vi "fxpProperty_OverflowModeDisabled_Write.vi"(4 "error in (no error)":errorcluster, 5 "Value":bool, 6 "Container State":T7, 7 "Display State In":T1) -> (0 "error out":errorcluster, 3 "Display State Out":T1)   [LabVIEW 2020, in "FXP.xctl"]
uses:
  <vilib>/fxp/FXPxcontrol/FXP.xctl
  <vilib>/_xctls/Container State.ctl
  <vilib>/fxp/FXPxcontrol/fxpState.ctl
  <vilib>/fxp/LVFixedPointQuantizationPolicyTypeDef.ctl
  <vilib>/fxp/LVFixedPointOverflowPolicyTypeDef.ctl
  <vilib>/fxp/FXPxcontrol/fxpChangeEvent.ctl
  <vilib>/fxp/FXPxcontrol/fxpValueChangeControl.ctl
  <vilib>/fxp/FXPxcontrol/fxpMixedStateStatus.ctl
  <vilib>/_xctls/XControlSupport.lvlib
panel:
  # "Replace the Value Control below with a Control of desired type.\nDo not remove this Control or the others from the connector pane.\nDo not change the connector pane pattern.\nThe Value control should always be the third terminal from top on the input side in the connector pane."
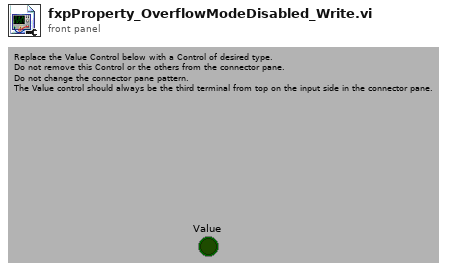
[diagram p1: front panel]
types:
  T1 = typedef "FXP.xctl/fxpState.ctl" = cluster{"disableAllConfig":bool, "disableEncodingConfig":bool, "disableRangeConfig":bool, "disableOverflowStatus":bool, "disableOverflowMode":bool, "visibleModes":bool, "visibleOverflowStatus":bool, "quantizationPolicy":T2, "overflowPolicy":T3, "includeOverflowStatus":bool, "changeEvent":T4, "valueChanged":T5, "mixed state":T6, "disableRoundingMode":bool}
  T2 = typedef "LVFixedPointQuantizationPolicyTypeDef.ctl" = enum32{"Truncate", "Round-Half-Up (Asymmetric)", "Round-Half-Even"}
  T3 = typedef "LVFixedPointOverflowPolicyTypeDef.ctl" = enum32{"Wrap", "Saturate"}
  T4 = typedef "FXP.xctl/fxpChangeEvent.ctl" = enum16{"<none>", "initialize", "modesVisible", "overflowModeEnabled", "overflowStatusVisible", "configEnabled", "modeRounding", "modeOverflow", "statusOverflow", "mixedState", "roundingModeEnabled"}
  T5 = typedef "FXP.xctl/fxpValueChangeControl.ctl" = enum16{"<none>", "sign", "word length", "integer word length", "minimum", "maximum", "delta", "rounding mode", "overflow mode", "overflow status"}
  T6 = typedef "FXP.xctl/fxpMixedStateStatus.ctl" = cluster{"sign":bool, "word length":bool, "integer word length":bool, "minimum":bool, "maximum":bool, "delta":bool, "rounding mode":bool, "overflow mode":bool, "overflow status":bool}
  T7 = typedef "XControlSupport.lvlib/Container State.ctl" = cluster{"Indicator?":bool, "Run Mode?":bool, " Refnum":refnum<vi>}
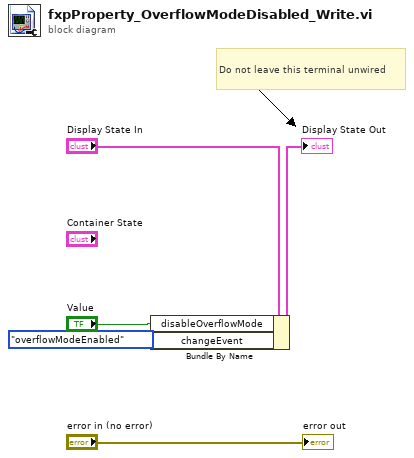
[diagram p0: block diagram]
diagram:
  # "Do not leave this terminal unwired"
  n1 = Bundle By Name(cluster="Display State In", "disableOverflowMode"="Value", "changeEvent"=fxpChangeEvent."overflowModeEnabled") -> (→"Display State Out":T1)
  "error out" <- "error in (no error)"
